vi "Array info.vi"(8 "error in (no error)":errorcluster, 11 "Variant":variant) -> (0 "error out":errorcluster, 2 "elements":variant[](array[variant]), 3 "child strings":string[](array[string]))   [LabVIEW 2017, in "DSF Configuration Utility.lvlib"]
uses:
  DSF Configuration Utility.lvlib
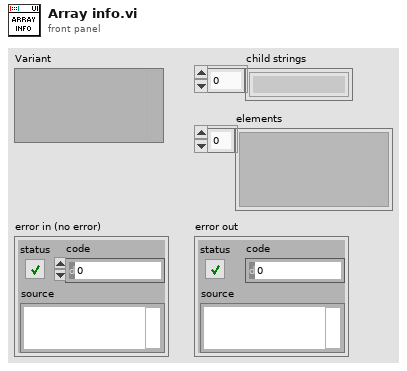
[diagram p1: front panel]
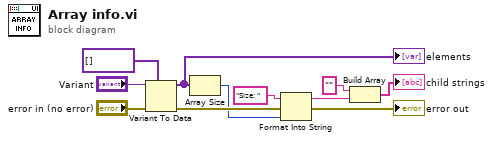
[diagram p0: block diagram]
diagram:
  n1 = Variant To Data(error in="error in (no error)", type=variant[] [], Variant="Variant") -> (data=w6:variant[], error out=w10:errorcluster)
  "elements" <- w6
  n2 = Array Size(array=w6) -> (size(s)=w7:i32)
  n3 = Format Into String(initial string="Size: " ("string"), error in=w10, w7) -> (resulting string=w3:string, error out=→"error out":errorcluster)  [unwired: 1 in]
  n4 = Build Array("" ("element"), w3) -> (→"child strings":string[])
